vi "DestroyTexture.vi"(8 "No Error":errorcluster, 11 "Texture [SDL_Texture *]":i64) -> (0 "error out":errorcluster)   [LabVIEW 2024, in "SDL3.lvlib" / "Render.lvlib"]
doc: "<B>Summary</B>\nDestroy the specified texture.\n\n<B>Remarks</B>\nPassing NULL or an otherwise invalid texture will set the SDL error message to \"Invalid texture\".\n\n<B>Thread Safety</B>\nYou may only call this function from the main thread."
uses:
  Render.lvlib
  Lib/SDL3-32.dll
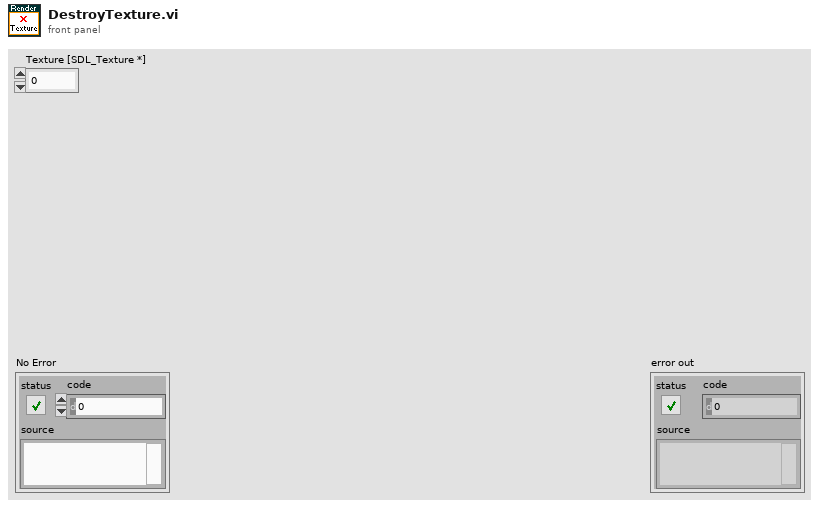
[diagram p1: front panel]
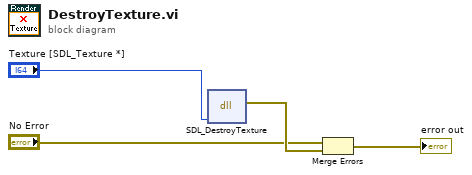
[diagram p0: block diagram]
diagram:
  n1 = dll-call lib="C:/Users/Thomas/Documents/Projects/LV-SDL3/Lib/SDL3-*.*" fn="SDL_DestroyTexture"("window"="Texture [SDL_Texture *]") -> (error out=w4:errorcluster)  [unwired: 5 in, 1 out]
  n2 = Merge Errors("No Error", w4) -> (→"error out":errorcluster)
